vi "TireBalancing.vi"() -> ()   [LabVIEW 2021]
uses:
  <vilib>/numeric/Random Number (Range) U64.vi
  <vilib>/numeric/sub_Random U32.vi
panel:
  out "x > y? 4":bool
  out "x > y? 3":bool
  out "x > y? 2":bool
  out "x > y?":bool
  in  "stop":bool
  in  "Play Button":bool
  in  "String 4":string
  in  "String 3":string
  in  "String 2":string
  in  "String":string
  out "s? t:f 4":string
  out "appended array 4":u64[](array[numeric])
  out "x = y? 4":bool[](array[boolean])
  out "s? t:f 3":string
  out "appended array 3":u64[](array[numeric])
  out "x = y? 3":bool[](array[boolean])
  out "s? t:f 2":string
  out "appended array 2":u64[](array[numeric])
  out "x = y? 2":bool[](array[boolean])
  out "s? t:f":string
  out "appended array":u64[](array[numeric])
  out "x = y?":bool[](array[boolean])
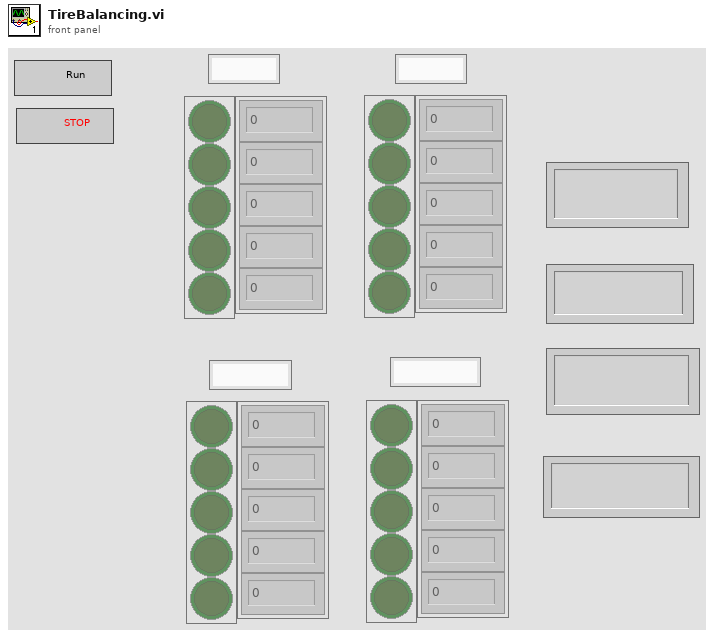
[diagram p1: front panel]
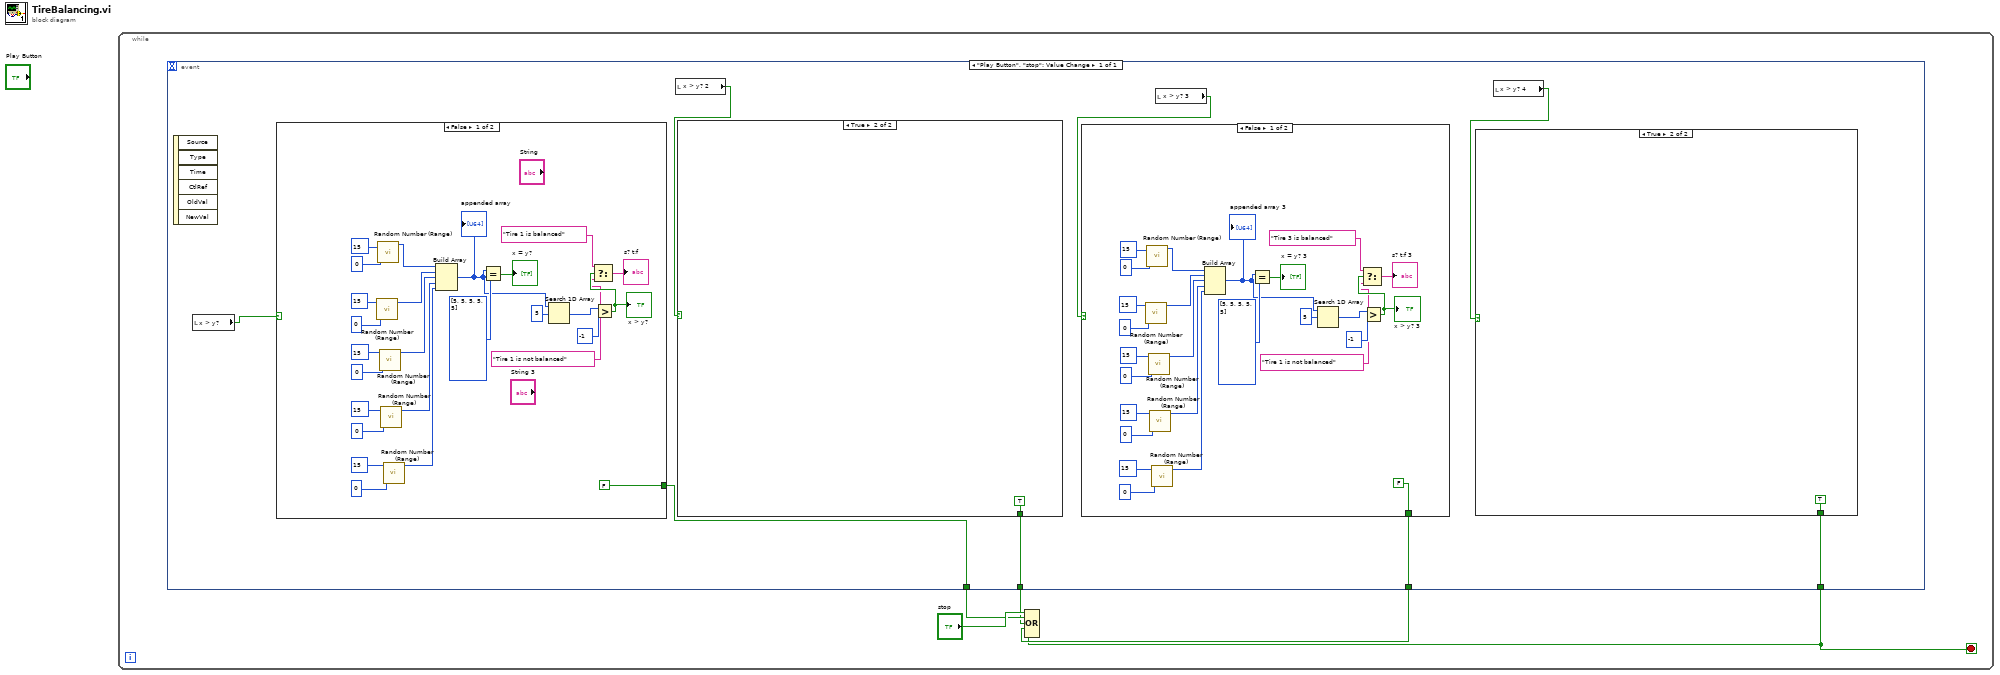
[diagram p0: block diagram]
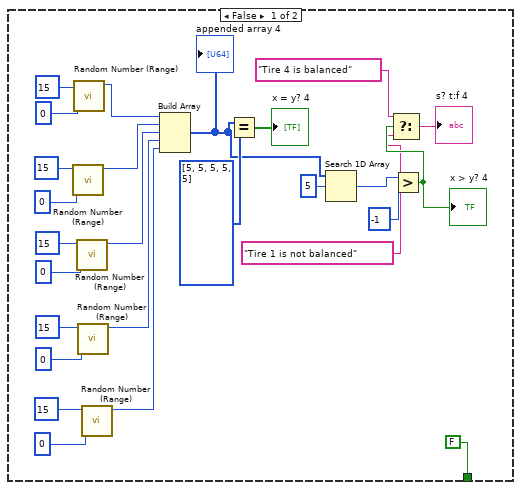
[diagram p2: hidden frame]
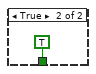
[diagram p3: hidden frame]
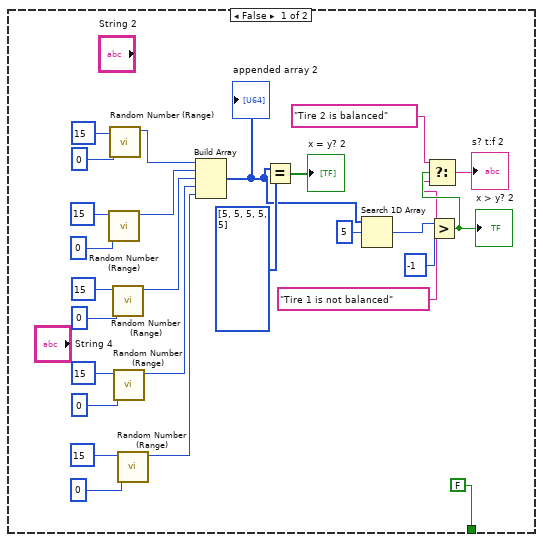
[diagram p4: hidden frame]
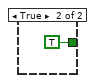
[diagram p5: hidden frame]
diagram:
  n1 = while {
    stop <- w1 stop-if-true
    n2 = event shown="[0] \"Play Button\", \"stop\": Value Change" {
      selector: _ -> [_]
      dyn-events: _ -> [_]
      timeout: _ -> [_]
      tunnel: [w12] -> w4
      tunnel: [w11] -> w3
      tunnel: [w10] -> w2
      tunnel: [w9] -> w1
      event "Play Button", "stop": Value Change {
        n3 = event-data() -> ()  [unwired: 1 in, 6 out]
        n4 = local read "x > y?"() -> (w13:bool)
        n5 = case shown="False" w13 {
          tunnel: [FALSE TRUE] -> w12
          frame False {
            n6 = call-poly <vilib>:"Random Number (Range).vi"("lower bound (0)"=u64 0, "upper bound (100)"=u64 15) -> ("number"=w109:u64)  [unwired: 9 in]
            n7 = call-poly <vilib>:"Random Number (Range).vi"("lower bound (0)"=u64 0, "upper bound (100)"=u64 15) -> ("number"=w110:u64)  [unwired: 9 in]
            n8 = call-poly <vilib>:"Random Number (Range).vi"("lower bound (0)"=u64 0, "upper bound (100)"=u64 15) -> ("number"=w108:u64)  [unwired: 9 in]
            n9 = call-poly <vilib>:"Random Number (Range).vi"("lower bound (0)"=u64 0, "upper bound (100)"=u64 15) -> ("number"=w107:u64)  [unwired: 9 in]
            n10 = call-poly <vilib>:"Random Number (Range).vi"("lower bound (0)"=u64 0, "upper bound (100)"=u64 15) -> ("number"=w106:u64)  [unwired: 9 in]
            n11 = Build Array(w110, w109, w108, w107, w106) -> (w103:u64[])
            "appended array" <- w103
            n12 = Equal?(x=w103, y=u64[] [5, 5, 5, 5, 5]) -> (x = y?=→"x = y?":bool[])
            n13 = Search 1D Array(1D array=w103, element=u64 5) -> (index of element=w101:i32)  [unwired: 1 in]
            n14 = Greater?(x=w101, y=-1) -> (0:w99:bool)
            "x > y?" <- w99
            n15 = Select(t="Tire 1 is balanced", s=w99, f="Tire 1 is not balanced") -> (s? t:f=→"s? t:f":string)
          }
          frame True {
          }
        }
        n16 = local read "x > y? 2"() -> (w8:bool)
        n17 = case shown="True" w8 {
          tunnel: [FALSE TRUE] -> w11
          frame False {
            n18 = call-poly <vilib>:"Random Number (Range).vi"("lower bound (0)"=u64 0, "upper bound (100)"=u64 15) -> ("number"=w82:u64)  [unwired: 9 in]
            n19 = call-poly <vilib>:"Random Number (Range).vi"("lower bound (0)"=u64 0, "upper bound (100)"=u64 15) -> ("number"=w83:u64)  [unwired: 9 in]
            n20 = call-poly <vilib>:"Random Number (Range).vi"("lower bound (0)"=u64 0, "upper bound (100)"=u64 15) -> ("number"=w81:u64)  [unwired: 9 in]
            n21 = call-poly <vilib>:"Random Number (Range).vi"("lower bound (0)"=u64 0, "upper bound (100)"=u64 15) -> ("number"=w80:u64)  [unwired: 9 in]
            n22 = call-poly <vilib>:"Random Number (Range).vi"("lower bound (0)"=u64 0, "upper bound (100)"=u64 15) -> ("number"=w79:u64)  [unwired: 9 in]
            n23 = Build Array(w83, w82, w81, w80, w79) -> (w76:u64[])
            "appended array 2" <- w76
            n24 = Equal?(x=w76, y=u64[] [5, 5, 5, 5, 5]) -> (x = y?=→"x = y? 2":bool[])
            n25 = Search 1D Array(1D array=w76, element=u64 5) -> (index of element=w74:i32)  [unwired: 1 in]
            n26 = Greater?(x=w74, y=-1) -> (0:w72:bool)
            "x > y? 2" <- w72
            n27 = Select(t="Tire 2 is balanced", s=w72, f="Tire 1 is not balanced") -> (s? t:f=→"s? t:f 2":string)
          }
          frame True {
          }
        }
        n28 = local read "x > y? 3"() -> (w7:bool)
        n29 = case shown="False" w7 {
          tunnel: [FALSE TRUE] -> w10
          frame False {
            n30 = call-poly <vilib>:"Random Number (Range).vi"("lower bound (0)"=u64 0, "upper bound (100)"=u64 15) -> ("number"=w55:u64)  [unwired: 9 in]
            n31 = call-poly <vilib>:"Random Number (Range).vi"("lower bound (0)"=u64 0, "upper bound (100)"=u64 15) -> ("number"=w56:u64)  [unwired: 9 in]
            n32 = call-poly <vilib>:"Random Number (Range).vi"("lower bound (0)"=u64 0, "upper bound (100)"=u64 15) -> ("number"=w54:u64)  [unwired: 9 in]
            n33 = call-poly <vilib>:"Random Number (Range).vi"("lower bound (0)"=u64 0, "upper bound (100)"=u64 15) -> ("number"=w53:u64)  [unwired: 9 in]
            n34 = call-poly <vilib>:"Random Number (Range).vi"("lower bound (0)"=u64 0, "upper bound (100)"=u64 15) -> ("number"=w52:u64)  [unwired: 9 in]
            n35 = Build Array(w56, w55, w54, w53, w52) -> (w49:u64[])
            "appended array 3" <- w49
            n36 = Equal?(x=w49, y=u64[] [5, 5, 5, 5, 5]) -> (x = y?=→"x = y? 3":bool[])
            n37 = Search 1D Array(1D array=w49, element=u64 5) -> (index of element=w47:i32)  [unwired: 1 in]
            n38 = Greater?(x=w47, y=-1) -> (0:w45:bool)
            "x > y? 3" <- w45
            n39 = Select(t="Tire 3 is balanced", s=w45, f="Tire 1 is not balanced") -> (s? t:f=→"s? t:f 3":string)
          }
          frame True {
          }
        }
        n40 = local read "x > y? 4"() -> (w6:bool)
        n41 = case shown="True" w6 {
          tunnel: [FALSE TRUE] -> w9
          frame False {
            n42 = call-poly <vilib>:"Random Number (Range).vi"("lower bound (0)"=u64 0, "upper bound (100)"=u64 15) -> ("number"=w28:u64)  [unwired: 9 in]
            n43 = call-poly <vilib>:"Random Number (Range).vi"("lower bound (0)"=u64 0, "upper bound (100)"=u64 15) -> ("number"=w29:u64)  [unwired: 9 in]
            n44 = call-poly <vilib>:"Random Number (Range).vi"("lower bound (0)"=u64 0, "upper bound (100)"=u64 15) -> ("number"=w27:u64)  [unwired: 9 in]
            n45 = call-poly <vilib>:"Random Number (Range).vi"("lower bound (0)"=u64 0, "upper bound (100)"=u64 15) -> ("number"=w26:u64)  [unwired: 9 in]
            n46 = call-poly <vilib>:"Random Number (Range).vi"("lower bound (0)"=u64 0, "upper bound (100)"=u64 15) -> ("number"=w25:u64)  [unwired: 9 in]
            n47 = Build Array(w29, w28, w27, w26, w25) -> (w22:u64[])
            "appended array 4" <- w22
            n48 = Equal?(x=w22, y=u64[] [5, 5, 5, 5, 5]) -> (x = y?=→"x = y? 4":bool[])
            n49 = Search 1D Array(1D array=w22, element=u64 5) -> (index of element=w20:i32)  [unwired: 1 in]
            n50 = Greater?(x=w20, y=-1) -> (0:w18:bool)
            "x > y? 4" <- w18
            n51 = Select(t="Tire 4 is balanced", s=w18, f="Tire 1 is not balanced") -> (s? t:f=→"s? t:f 4":string)
          }
          frame True {
          }
        }
      }
    }
    n52 = Compound Arithmetic op=OR("stop", w4, w3, w2, w1) -> ()  [unwired: 1 out]
  }
